vi "create missing folders.vi"(8 "error in (no error)":errorcluster, 10 "path":path, 11 "TomoConversion in":refnum<class "TomoConversion.lvclass">) -> (0 "error out":errorcluster, 3 "TomoConversion out":refnum<class "TomoConversion.lvclass">)   [LabVIEW 2012, in "TomoConversion.lvclass"]
uses:
  TomoConversion.lvclass
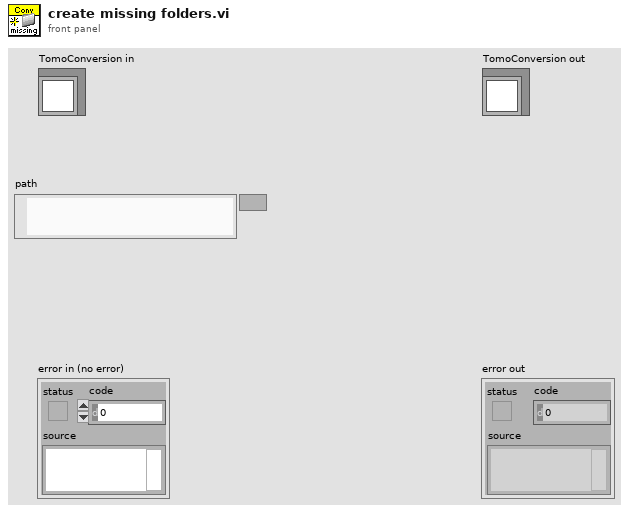
[diagram p1: front panel]
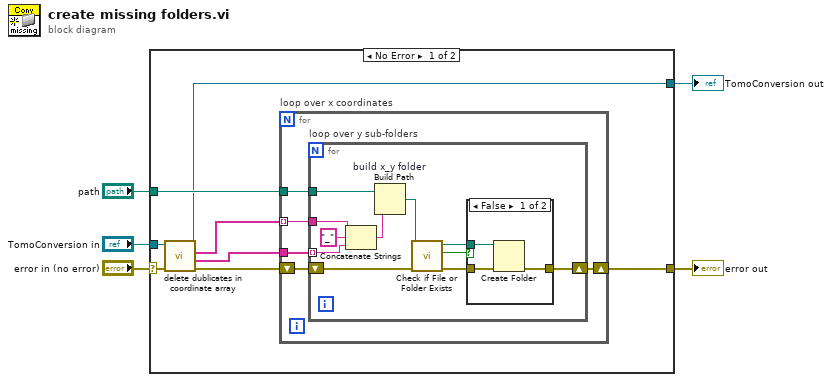
[diagram p0: block diagram]
diagram:
  n1 = case shown="No Error" "error in (no error)" {
    selector: "error in (no error)" -> [w13 w35]
    tunnel: [w7 w35] -> w4
    tunnel: [w6 w34] -> w2
    tunnel: "TomoConversion in" -> [w11 w34]
    tunnel: "path" -> [w9 _]
    frame No Error {
      n2 = call-dynamic "delete dublicates in coordinate array.vi"("error in (no error)"=w13, "TomoConversion in"=w11) -> ("error out"=w10:errorcluster, "y coordinate array"=w8:string[], "x coordinate array"=w12:string[], "TomoConversion out"=w6:refnum<class "TomoConversion.lvclass">)  [unwired: 6 in]
      n3 = for "loop over x coordinates" {
        tunnel: w12 -> [w16] mode=indexing
        shift-right: [w14] -> w7
        shift-left: w10 -> [w18]
        tunnel: w9 -> [w17]
        tunnel: w8 -> [w15]
        n4 = for "loop over y sub-folders" {
          tunnel: w17 -> [w25]
          tunnel: w16 -> [w23]
          tunnel: w15 -> [w21] mode=indexing
          shift-right: [w19] -> w14
          shift-left: w18 -> [w26]
          n5 = Concatenate Strings(w23, "_" ("string"), w21) -> (w22:string)
          n6 = Build Path "build x_y folder"(base path=w25, name or relative path=w22) -> (appended path=w20:path)
          n7 = call <vilib>:"Check if File or Folder Exists.vi"("error in (no error)"=w26, "path"=w20) -> ("error out"=w28:errorcluster, "file or folder exists?"=w27:bool, "dup path"=w29:path)  [unwired: 7 in]
          n8 = case shown="False" w27 {
            tunnel: w28 -> [w32 w33]
            tunnel: [w31 w33] -> w19
            tunnel: w29 -> [w30 _]
            frame False {
              n9 = Create Folder(path (use dialog)=w30, error in=w32) -> (error out=w31:errorcluster)  [unwired: 1 in, 2 out]
            }
            frame True {
            }
          }
        }
      }
    }
    frame Error {
    }
  }
  "error out" <- w4
  "TomoConversion out" <- w2
